vi "Add VI Icon Layer.vi"(8 "error in (no error)":errorcluster, 11 "VI Ref":refnum<vi>) -> (0 "error out":errorcluster, 2 "Save?":bool, 3 "VI Ref out":refnum<vi>)   [LabVIEW 2020, in "Code Cleanup.lvlib"]
uses:
  Code Cleanup.lvlib
  <vilib>/LabVIEW Icon API/lv_icon/Classes/Layer/Layer.lvclass
  <vilib>/LabVIEW Icon API/lv_icon/Classes/Icon/Icon.lvclass
  <vilib>/LabVIEW Icon API/lv_icon/Classes/Icon Framework/Icon Framework.lvclass
  <vilib>/LabVIEW Icon API/lv_icon/Controls/LayerType.ctl
  <vilib>/LabVIEW Icon API/lv_icon/Controls/Layer.ctl
  <vilib>/LabVIEW Icon API/LabVIEW Icon API.lvlib
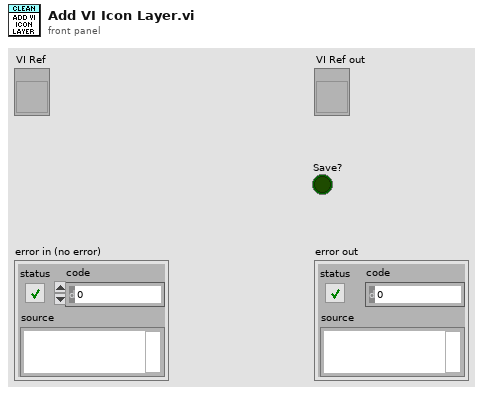
[diagram p1: front panel]
types:
  T1 = cluster{"left":i16, "top":i16, "right":i16, "bottom":i16}
  T2 = typedef "Layer.ctl" = cluster{"LayerIcon":picture, "LayerName":string, "Opacity":u8, "Visibility?":bool}
  T3 = typedef "LayerType.ctl" = enum16{"Graphic", "Text", "Tool", "Graphic Drop"}
  T4 = typedef "imagedata.ctl" = cluster{"image type":i32, "image depth":i32, "image":u8[], "mask":u8[], "colors":u32[], "Rectangle":cluster{"left":i16, "top":i16, "right":i16, "bottom":i16}}
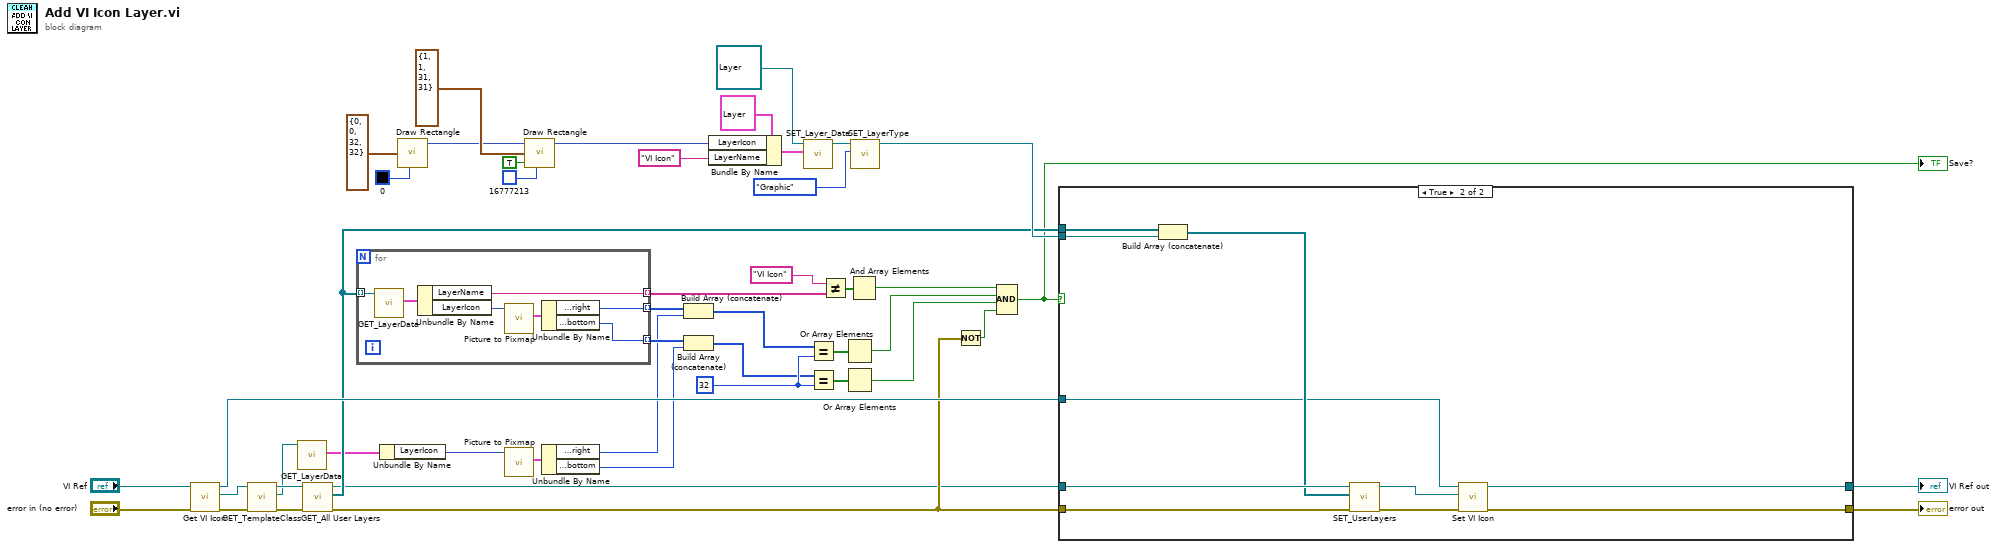
[diagram p0: block diagram]
diagram:
  w43 = i16 32 ("x")
  n1 = call <vilib>:"Get VI Icon.vi"("error in (no error)"="error in (no error)", "VI Refnum in"="VI Ref") -> ("error out"=w18:errorcluster, "Icon"=w16:refnum<class "Icon.lvclass">, "VI Refnum out"=w25:refnum<vi>)  [unwired: 7 in]
  n2 = call-dynamic "GET_TemplateClass.vi"("error in (no error)"=w18, "Icon.lvclass in"=w16) -> ("error out"=w17:errorcluster, "Icon Framework.lvclass"=w14:refnum<class "Icon Framework.lvclass">, "Icon.lvclass out"=w15:refnum<class "Icon.lvclass">)  [unwired: 7 in]
  n3 = call-dynamic "GET_LayerData.vi"("Layer.lvclass in"=w14) -> ("Data"=w13:T2)  [unwired: 6 in, 4 out]
  n4 = call-dynamic "GET_All User Layers.vi"("error in (no error)"=w17, "Icon.lvclass in"=w15) -> ("error out"=w23:errorcluster, "User Layer"=w24:refnum<class "Layer.lvclass">[], "Icon.lvclass out"=w22:refnum<class "Icon.lvclass">)  [unwired: 7 in]
  n5 = for {
    tunnel: w24 -> [w53] mode=indexing
    tunnel: [w52] -> w46 mode=indexing
    tunnel: [w49] -> w9 mode=indexing
    tunnel: [w48] -> w8 mode=indexing
    n6 = call-dynamic "GET_LayerData.vi"("Layer.lvclass in"=w53) -> ("Data"=w54:T2)  [unwired: 6 in, 4 out]
    n7 = Unbundle By Name(w54) -> ("LayerName"=w52:string, "LayerIcon"=w51:picture)
    n8 = call <vilib>:"Picture to Pixmap.vi"("picture"=w51) -> ("image data"=w50:T4)  [unwired: 9 in, 1 out]
    n9 = Unbundle By Name(w50) -> ("Rectangle.right"=w49:i16, "Rectangle.bottom"=w48:i16)
  }
  n10 = Unbundle By Name(w13) -> ("LayerIcon"=w11:picture)
  n11 = call <vilib>:"Draw Rectangle.vi"("rect"=T1 {"left"=0, "top"=0, "right"=32, "bottom"=32}, "color(black)"=u32 0) -> ("new picture"=w33:picture)  [unwired: 7 in]
  n12 = call <vilib>:"Picture to Pixmap.vi"("picture"=w11) -> ("image data"=w12:T4)  [unwired: 9 in, 1 out]
  n13 = call <vilib>:"Draw Rectangle.vi"("picture"=w33, "rect"=T1 {"left"=1, "top"=1, "right"=31, "bottom"=31}, "fill?(F)"=TRUE, "color(black)"=u32 16777213) -> ("new picture"=w29:picture)  [unwired: 5 in]
  n14 = Unbundle By Name(w12) -> ("Rectangle.right"=w7:i16, "Rectangle.bottom"=w6:i16)
  n15 = Build Array (concatenate)(w9, w7) -> (w5:i16[])
  n16 = Build Array (concatenate)(w8, w6) -> (w4:i16[])
  n17 = Bundle By Name(cluster=T2 {"LayerIcon"=bytes[3102], "LayerName"="", "Opacity"=100, "Visibility?"=TRUE} ("Data"), "LayerIcon"=w29, "LayerName"="VI Icon") -> (w28:T2)
  n18 = call-dynamic "SET_Layer_Data.vi"("Data"=w28, "Layer.lvclass in"=refnum<class "Layer.lvclass"> refnum) -> ("Layer.lvclass out"=w30:refnum<class "Layer.lvclass">)  [unwired: 8 in, 1 out]
  n19 = Equal?(x=w5, y=w43) -> (x = y?=w42:bool[])
  n20 = Equal?(x=w4, y=w43) -> (x = y?=w41:bool[])
  n21 = Not Equal?(x="VI Icon", y=w46) -> (x != y?=w45:bool[])
  n22 = Or Array Elements(Boolean array=w42) -> (logical OR=w20:bool)
  n23 = Or Array Elements(Boolean array=w41) -> (logical OR=w19:bool)
  n24 = And Array Elements(Boolean array=w45) -> (logical AND=w44:bool)
  n25 = call-dynamic "SET_LayerType.vi"("Type"=LayerType."Graphic", "Layer.lvclass in"=w30) -> ("Layer.lvclass out"=w27:refnum<class "Layer.lvclass">)  [unwired: 8 in, 1 out]
  n26 = Not(x=w23) -> (.not. x?=w40:bool)
  n27 = Compound Arithmetic op=AND(w44, w20, w19, w40) -> (w2:bool)
  "Save?" <- w2
  n28 = case shown="True" w2 {
    tunnel: w23 -> [w56 w64]
    tunnel: [w56 w58] -> w47
    tunnel: [w55 w57] -> w1
    tunnel: w25 -> [w55 w59]
    tunnel: w24 -> [_ w66]
    tunnel: w27 -> [_ w65]
    tunnel: w22 -> [_ w63]
    frame False {
    }
    frame True {
      n29 = Build Array (concatenate)(w66, w65) -> (w62:refnum<class "Layer.lvclass">[])
      n30 = call-dynamic "SET_UserLayers.vi"("error in (no error)"=w64, "Layers"=w62, "Icon.lvclass in"=w63) -> ("error out"=w61:errorcluster, "Icon.lvclass out"=w60:refnum<class "Icon.lvclass">)  [unwired: 7 in]
      n31 = call <vilib>:"Set VI Icon.vi"("error in (no error)"=w61, "Icon"=w60, "VI Refnum in"=w59) -> ("error out"=w58:errorcluster, "VI Refnum out"=w57:refnum<vi>)  [unwired: 7 in]
    }
  }
  "error out" <- w47
  "VI Ref out" <- w1
